vi "CRYFreq or Log Amp Sweep.vi"(4 "Output Flag":cluster{bool, bool, "ApplyEQ":bool}, 6 "Stimulus Para":T3={"Name"="", "Level Out"=0.9999999999999998, "Start Freq"=6300.0, "Stop Freq"=100.0, "Steps"=19, "Cycles"=12, "Sweep type"=0, "Freq"=1000.0, "Start ampl"=0.9999999999999998, "Stop ampl"=0.9999999999999998, "sine waves"=[], "wav path"="", "Sweep time"=0.9999999999999998, "Resolution"=0, "Tone type6"=0, "fix/ratio6"=0, "Ratio6"=0, "Difference6"=0, "RatioFreq6"=0} {"Resolution" items=["R10(1/3 Oct.)", "R20(1/6 Oct.)", "R40(1/12 Oct.)", "R80(1/24 Oct.)", "User Defined, Log", "User Defined,Linear"]; "Sweep time" format="%.2f"; "Stop ampl" format="%.2f"; "Start ampl" format="%.2f"; "Freq" format="%.2f"; "sine waves"."cycles" format="%.2f"; "sine waves"."ampl" format="%.2f"; "sine waves"."freq" format="%.2f"; "Level Out" format="%.2f"}, 7 "end":bool, 8 "FAPS in":T4(array[cluster]) {"cycles" format="%.2f"; "ampl" format="%.2f"; "freq" format="%.2f"}, 9 "Master sine waves":cluster{"freq":dbl, "ampl":dbl, "cycles":dbl}[](array[cluster]) {"cycles" format="%.2f"; "ampl" format="%.2p"; "freq" format="%.2f"}, 10 "EQ Curve":T1={"Name"="", "Curve"=[], "X data"=1, "Y data"=1, "Z data"=1, "X axis"=0, "Y axis"=1, "Z axis"=1, "X unit"="Hz", "Y unit"="", "Z unit"="deg.", "X dB ref"=1.0, "Y dB ref"=1.0, "Z dB ref"=1.0, "single val"=FALSE, "protected"=FALSE, "display X"=TRUE, "display Y"=TRUE, "display Z"=TRUE, "Test Info"="", "Step No."=0, "Plot Settings"={"Color"=0, "Interpolation"=0, "Point Style"=0, "Line Style"=0, "Point Color"=0, "Line Width"=0, "Bar Plot Style"=0, "Fill To"=0}, "AutoProtect"=FALSE} {"Z data" items=["dB", "Lin"]; "X data" items=["dB", "Lin"]; "Y data" items=["dB", "Lin"]; "Z dB ref" format="%.1f"; "Z axis" items=["Log", "Lin"]; "X dB ref" format="%.1f"; "X axis" items=["Log", "Lin"]; "Y axis" items=["Log", "Lin"]; "Y dB ref" format="%.1f"; "Curve"."z" format="%.2f"; "Curve"."y" format="%.2f"; "Curve"."x" format="%.2f"}, 11 "Param1":T2) -> (1 "FAPS out":T4(array[cluster]) {"cycles" format="%.2f"; "ampl" format="%.2f"; "freq" format="%.2f"}, 2 "Stimulus out":sgl[](array[numeric]), 3 "Diff Frequency":dbl)   [LabVIEW 2013]
uses:
  Typedef Control/CRYStimulus Parameter.ctl
  Typedef Control/CRYData Cluster.ctl
  <vilib>/Analysis/NI_AALBase.lvlib
panel:
  out "x/y":dbl format="%#_6p"
  out "Waveform Graph":waveform(sgl)(graph)
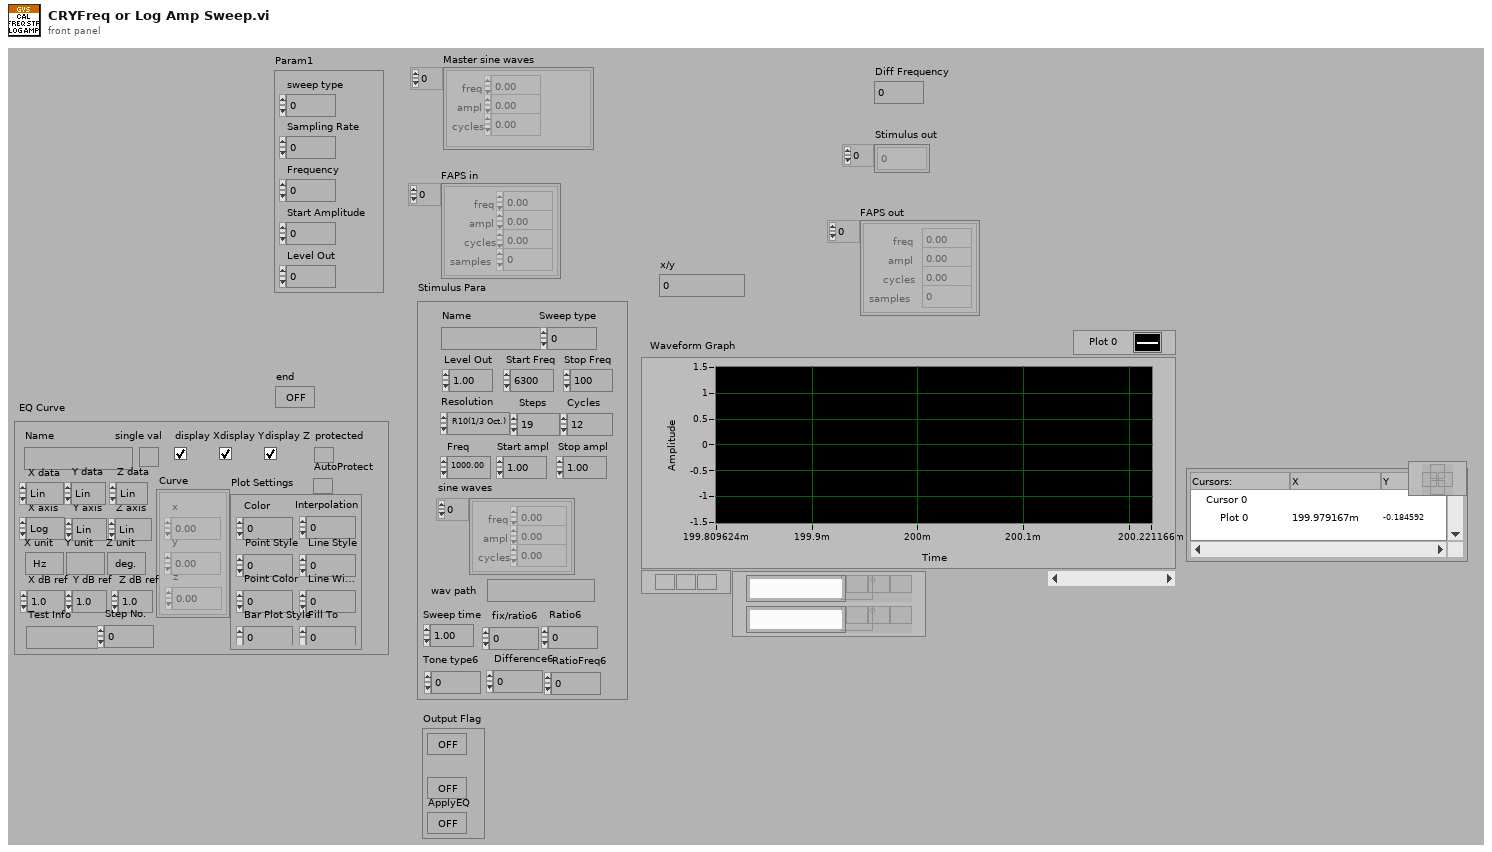
[diagram p1: front panel]
types:
  T1 = typedef "CRYData Cluster.ctl" = cluster{"Name":string, "Curve":cluster{"x":dbl, "y":dbl, "z":dbl}[], "X data":u16, "Y data":u16, "Z data":u16, "X axis":u16, "Y axis":u16, "Z axis":u16, "X unit":string, "Y unit":string, "Z unit":string, "X dB ref":dbl, "Y dB ref":dbl, "Z dB ref":dbl, "single val":bool, "protected":bool, "display X":bool, "display Y":bool, "display Z":bool, "Test Info":string, "Step No.":i32, "Plot Settings":cluster{"Color":u32, "Interpolation":u8, "Point Style":u8, "Line Style":u8, "Point Color":u32, "Line Width":u8, "Bar Plot Style":u8, "Fill To":i16}, "AutoProtect":bool}
  T2 = cluster{"sweep type":i32, "Sampling Rate":dbl, "Frequency":dbl, "Start Amplitude":dbl, "Level Out":dbl}
  T3 = typedef "CRYStimulus Parameter.ctl" = cluster{"Name":string, "Level Out":dbl, "Start Freq":dbl, "Stop Freq":dbl, "Steps":u32, "Cycles":u32, "Sweep type":i32, "Freq":dbl, "Start ampl":dbl, "Stop ampl":dbl, "sine waves":cluster{"freq":dbl, "ampl":dbl, "cycles":dbl}[], "wav path":string, "Sweep time":dbl, "Resolution":u16, "Tone type6":u16, "fix/ratio6":u16, "Ratio6":u16, "Difference6":u32, "RatioFreq6":u32}
  T4 = cluster{"freq":dbl, "ampl":dbl, "cycles":dbl, "samples":i32}[]
  T5 = cluster{"freq":dbl, "ampl":dbl, "cycles":dbl, "samples":i32}
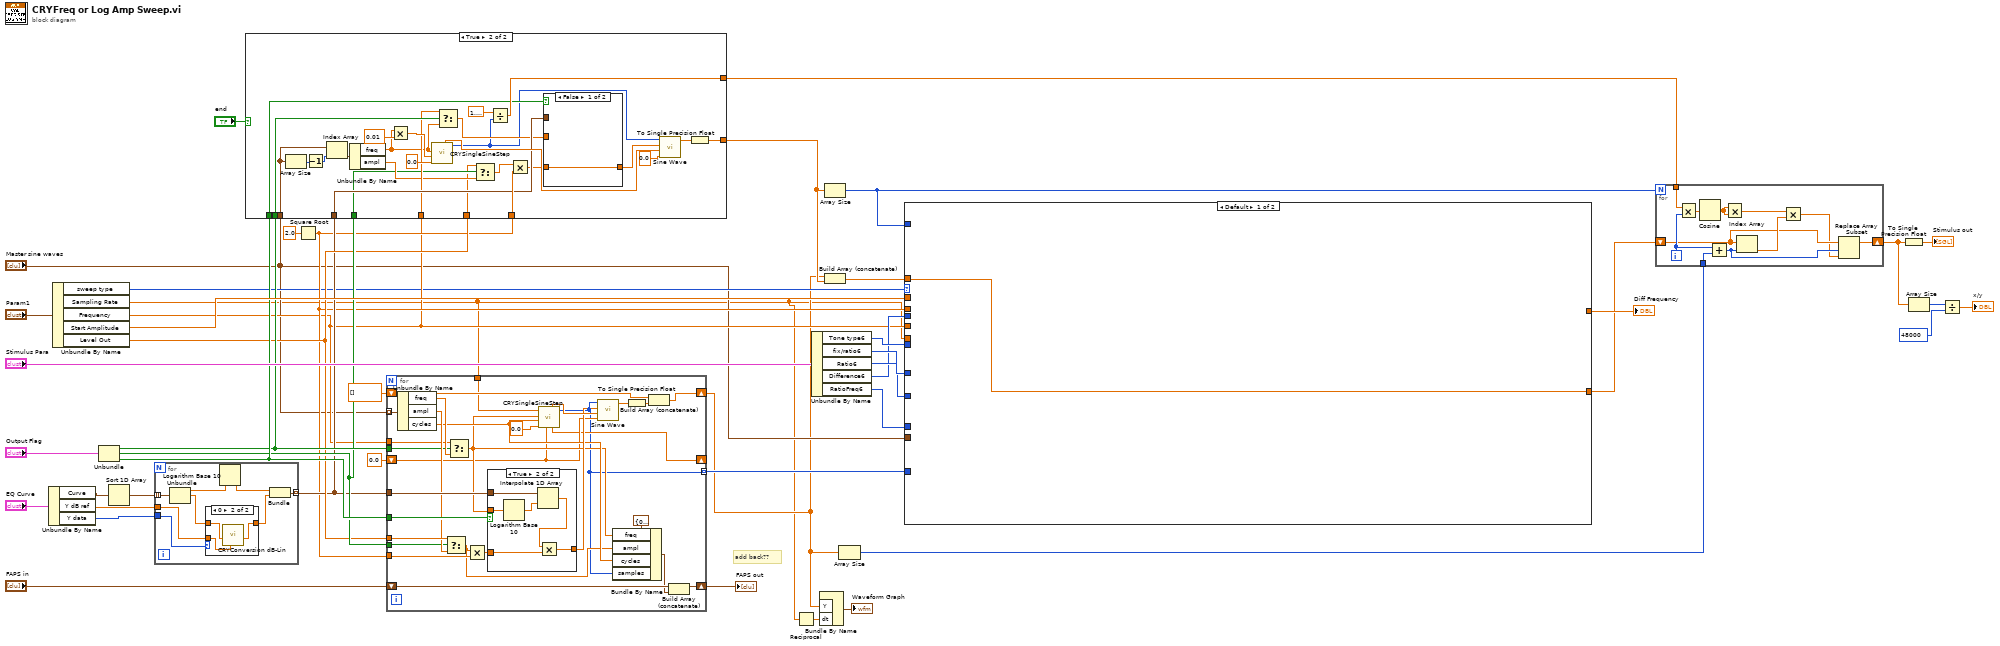
[diagram p0: block diagram]
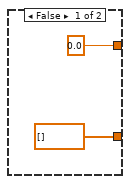
[diagram p2: hidden frame]
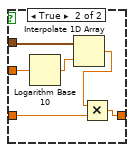
[diagram p3: hidden frame]
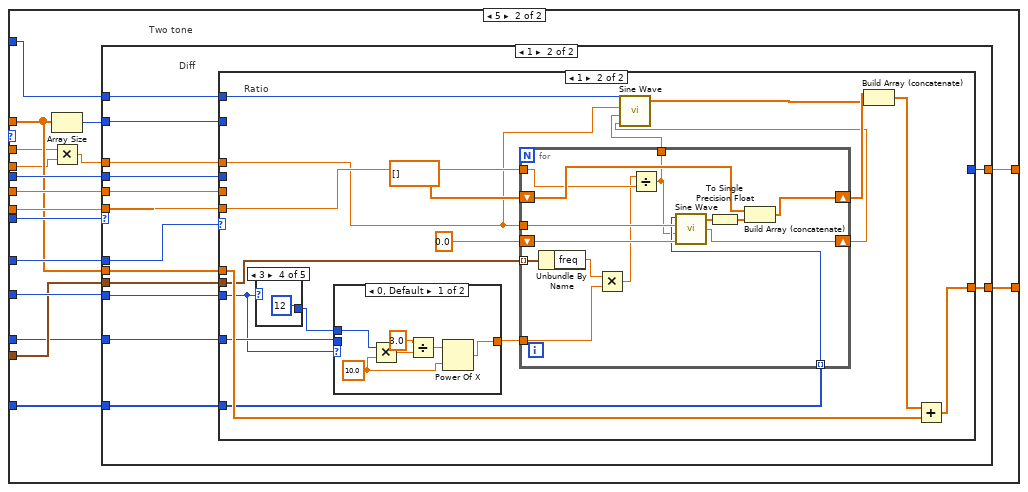
[diagram p6: hidden frame]
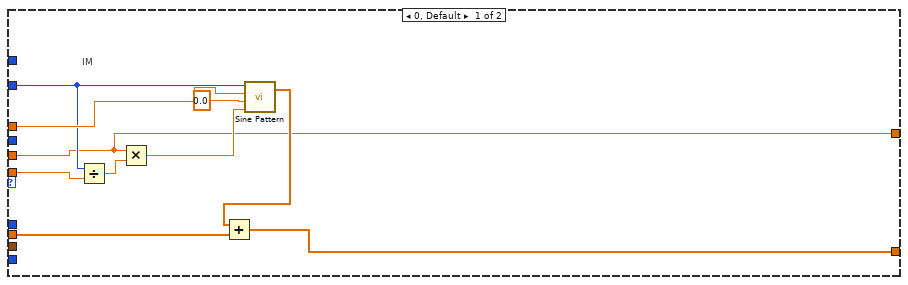
[diagram p7: hidden frame]
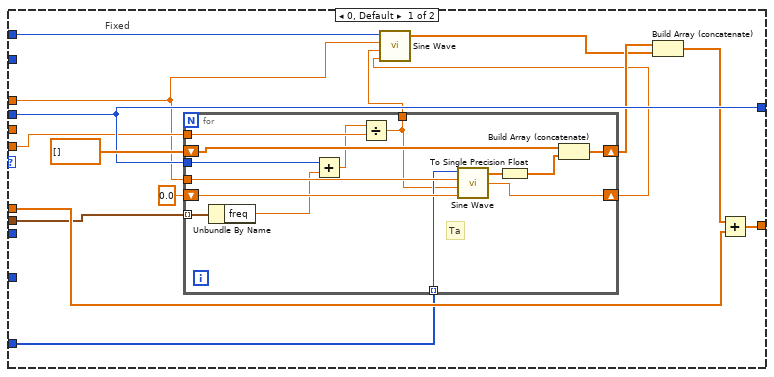
[diagram p8: hidden frame]
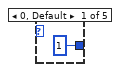
[diagram p9: hidden frame]
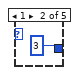
[diagram p10: hidden frame]
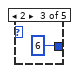
[diagram p11: hidden frame]
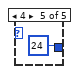
[diagram p12: hidden frame]
diagram:
  # "add back??"
  n1 = Unbundle By Name("EQ Curve") -> ("Curve"=w23:cluster{"x":dbl, "y":dbl, "z":dbl}[], "Y dB ref"=w22:dbl, "Y data"=w21:u16)
  n2 = Unbundle By Name("Param1") -> ("sweep type"=w10:i32, "Sampling Rate"=w6:dbl, "Frequency"=w13:dbl, "Start Amplitude"=w32:dbl, "Level Out"=w26:dbl)
  n3 = Unbundle("Output Flag") -> (w28:bool, w27:bool, "ApplyEQ"=w29:bool)
  n4 = Sort 1D Array(array=w23) -> (sorted array=w35:cluster{"x":dbl, "y":dbl, "z":dbl}[])
  n5 = for {
    tunnel: w35 -> [w54] mode=indexing
    tunnel: [w52] -> w20 mode=indexing
    tunnel: w22 -> [w50]
    tunnel: w21 -> [w49]
    n6 = Unbundle(w54) -> ("x"=w48:dbl, "y"=w47:dbl)  [unwired: 1 out]
    n7 = case shown="0" w49 {
      tunnel: w47 -> [w55 w58]
      tunnel: [w55 w57] -> w51
      tunnel: w50 -> [_ w56]
      frame 1, Default {
      }
      frame 0 {
        n8 = call "CRYConversion dB-Lin.vi"("dB ref."=w56, "Log In"=w58) -> ("Lin Out"=w57:dbl)  [unwired: 4 in, 3 out]
      }
    }
    n9 = Logarithm Base 10(1:w48) -> (0:w53:dbl)
    n10 = Bundle(w53, "Lin Out"=w51) -> (w52:cluster{dbl, "Lin Out":dbl})  [unwired: 1 out]
  }
  n11 = Square Root(x=2.0) -> (sqrt(x)=w14:dbl)
  n12 = case shown="True" "end" {
    tunnel: "Master sine waves" -> [_ w77]
    tunnel: [0.0 w76] -> w31
    tunnel: w14 -> [_ w75]
    tunnel: w29 -> [_ w74]
    tunnel: w20 -> [_ w73]
    tunnel: w28 -> [_ w72]
    tunnel: w13 -> [_ w70]
    tunnel: [sgl[] [] w69] -> w16
    tunnel: w27 -> [_ w64]
    tunnel: w26 -> [_ w63]
    frame False {
    }
    frame True {
      n13 = Array Size(array=w77) -> (size(s)=w87:i32)
      n14 = Decrement(x=w87) -> (x-1=w86:i32)
      n15 = Index Array(array=w77, index=w86) -> (element=w85:cluster{"freq":dbl, "ampl":dbl, "cycles":dbl})
      n16 = Unbundle By Name(w85) -> ("freq"=w61:dbl, "ampl"=w66:dbl)
      n17 = Multiply(x=w61, y=0.01) -> (x*y=w79:dbl)
      n18 = call "CRYSingleSineStep.vi"("Freq"=w61, "Cycles per freq"=w79, "Cycles discarded"=0.0) -> ("RelFreq"=w83:dbl, "TotalSamples"=w62:i32)  [unwired: 2 in, 4 out]
      n19 = Select(t=w70, s=w72, f=w61) -> (s? t:f=w71:dbl)
      n20 = Select(t=w63, s=w64, f=w66) -> (s? t:f=w65:dbl)
      n21 = Divide(x=1.5707963267948966, y=w62) -> (x/y=w76:dbl)
      n22 = Multiply(x=w65, y=w75) -> (x*y=w68:dbl)
      n23 = case shown="False" w74 {
        tunnel: [w88 w91] -> w67
        tunnel: w68 -> [w88 w94]
        tunnel: w73 -> [_ w92]
        tunnel: w71 -> [_ w89]
        frame False {
        }
        frame True {
          n24 = Logarithm Base 10(1:w89) -> (0:w90:dbl)
          n25 = Interpolate 1D Array(1:w90, 2:w92) -> (0:w93:dbl)
          n26 = Multiply(x=w93, y=w94) -> (x*y=w91:dbl)
        }
      }
      n27 = call <vilib>:"Sine Wave.vi"("samples"=w62, "amplitude"=w67, "frequency"=w83, "phase in"=0.0) -> ("sine wave"=w81:dbl[])  [unwired: 1 in, 2 out]
      n28 = To Single Precision Float(number=w81) -> (single precision float=w69:sgl[])
    }
  }
  n29 = for {
    shift-right: [w123] -> w8
    shift-left: sgl[] [] -> [w122]
    tunnel: w29 -> [w120]
    tunnel: w20 -> [w121]
    tunnel: "Master sine waves" -> [w119] mode=indexing
    tunnel: w14 -> [w118]
    tunnel: w6 -> [w110]
    tunnel: w26 -> [w116]
    tunnel: w13 -> [w111]
    shift-right: [w99] -> _
    shift-left: 0.0 -> [w100]
    shift-right: [w95] -> w39
    shift-left: "FAPS in" -> [w97]
    tunnel: w27 -> [w104]
    tunnel: w28 -> [w103]
    tunnel: [w98] -> w17 mode=indexing
    n30 = Unbundle By Name(w119) -> ("freq"=w115:dbl, "ampl"=w113:dbl, "cycles"=w106:dbl)
    n31 = Select(t=w116, s=w104, f=w113) -> (s? t:f=w102:dbl)
    n32 = Select(t=w111, s=w103, f=w115) -> (s? t:f=w101:dbl)
    n33 = Multiply(x=w102, y=w118) -> (x*y=w117:dbl)
    n34 = case shown="True" w120 {
      tunnel: [w124 w127] -> w107
      tunnel: w117 -> [w124 w130]
      tunnel: w121 -> [_ w128]
      tunnel: w101 -> [_ w126]
      frame False {
      }
      frame True {
        n35 = Logarithm Base 10(1:w126) -> (0:w125:dbl)
        n36 = Interpolate 1D Array(1:w125, 2:w128) -> (0:w129:dbl)
        n37 = Multiply(x=w129, y=w130) -> (x*y=w127:dbl)
      }
    }
    n38 = call "CRYSingleSineStep.vi"("Fs"=w110, "Freq"=w101, "Cycles per freq"=w106, "Cycles discarded"=0.0 ("phase in"), "StartPhase"=w100) -> ("RelFreq"=w108:dbl, "StopPhase"=w99:dbl, "TotalSamples"=w98:i32)  [unwired: 3 out]
    n39 = call <vilib>:"Sine Wave.vi"("samples"=w98, "amplitude"=w107, "frequency"=w108, "phase in"=w100) -> ("sine wave"=w114:dbl[])  [unwired: 1 in, 2 out]
    n40 = Bundle By Name(cluster=T5 {"freq"=0.0, "ampl"=0.0, "cycles"=0.0, "samples"=0}, "freq"=w101, "ampl"=w102, "cycles"=w106, "samples"=w98) -> (w96:T5)
    n41 = To Single Precision Float(number=w114) -> (single precision float=w109:sgl[])
    n42 = Build Array (concatenate)(w122, w109) -> (w123:sgl[])
    n43 = Build Array (concatenate)(w97, w96) -> (w95:T4)
  }
  "FAPS out" <- w39
  n44 = Reciprocal(x=w6) -> (1/x=w5:dbl)
  n45 = Unbundle By Name("Stimulus Para") -> ("Tone type6"=w46:u16, "fix/ratio6"=w45:u16, "Ratio6"=w44:u16, "Difference6"=w43:u32, "RatioFreq6"=w42:u32)
  n46 = Bundle By Name("Y"=w8, "dt"=w5) -> (→"Waveform Graph":waveform(sgl))  [unwired: 1 in]
  n47 = Build Array (concatenate)(w8, w16) -> (w19:sgl[])
  n48 = Array Size(array=w16) -> (size(s)=w18:i32)
  n49 = Array Size(array=w8) -> (size(s)=w30:i32)
  n50 = case shown="Default" w10 {
    tunnel: [w131 w148] -> w15
    tunnel: w43 -> [_ w142]
    tunnel: w46 -> [_ w147]
    tunnel: w45 -> [_ w146]
    tunnel: w44 -> [_ w145]
    tunnel: w6 -> [_ w144]
    tunnel: w13 -> [_ w143]
    tunnel: "Master sine waves" -> [_ w141]
    tunnel: w42 -> [_ w140]
    tunnel: [_ w139] -> w41
    tunnel: w19 -> [w131 w138]
    tunnel: w32 -> [_ w136]
    tunnel: w14 -> [_ w135]
    tunnel: w18 -> [_ w133]
    tunnel: w17 -> [_ w132]
    frame Default {
    }
    frame 5 {
      # "Two tone"
      n51 = Array Size(array=w138) -> (size(s)=w137:i32)
      n52 = Multiply(x=w136, y=w135) -> (x*y=w134:dbl)
      n53 = case shown="1" w147 {
        tunnel: w138 -> [w158 w172]
        tunnel: [w150 w171] -> w148
        tunnel: w137 -> [w153 w170]
        tunnel: w134 -> [w157 w169]
        tunnel: w146 -> [_ w168]
        tunnel: w145 -> [_ w167]
        tunnel: w144 -> [w151 w166]
        tunnel: w143 -> [w149 w165]
        tunnel: w142 -> [_ w164]
        tunnel: w141 -> [_ w159]
        tunnel: w140 -> [_ w163]
        tunnel: [w149 w162] -> w139
        tunnel: w133 -> [_ w161]
        tunnel: w132 -> [_ w160]
        frame 0, Default {
          # "IM"
          n54 = Divide(x=w153, y=w151) -> (x/y=w152:dbl)
          n55 = Multiply(x=w149, y=w152) -> (x*y=w154:dbl)
          n56 = call <vilib>:"Sine Pattern.vi"("cycles"=w154, "phase(degrees)"=0.0 ("phase in"), "amplitude"=w157, "samples"=w153) -> ("Sinusoidal Pattern"=w155:dbl[])  [unwired: 1 out]
          n57 = Add(x=w155, y=w158) -> (x+y=w150:dbl[])
        }
        frame 1 {
          # "Diff"
          n58 = case shown="1" w168 {
            tunnel: w172 -> [w185 w217]
            tunnel: [w176 w205] -> w171
            tunnel: w170 -> [_ _]
            tunnel: w169 -> [w175 w203]
            tunnel: w167 -> [_ w213]
            tunnel: w166 -> [w177 w210]
            tunnel: w165 -> [_ _]
            tunnel: w164 -> [w182 _]
            tunnel: w159 -> [w184 w204]
            tunnel: w163 -> [_ w214]
            tunnel: [w182 _] -> w162
            tunnel: w161 -> [w183 w209]
            tunnel: w160 -> [w180 w207]
            frame 0, Default {
              # "Fixed"
              n59 = for {
                tunnel: w175 -> [w201]
                tunnel: w184 -> [w200] mode=indexing
                shift-right: [w198] -> w174
                shift-left: 0.0 ("phase in") -> [w199]
                shift-right: [w195] -> w179
                shift-left: sgl[] [] -> [w196]
                tunnel: w182 -> [w197]
                tunnel: w177 -> [w192]
                tunnel: w180 -> [w189] mode=indexing
                tunnel: [w188] -> w173
                # "Ta"
                n60 = Unbundle By Name(w200) -> ("freq"=w191:dbl)
                n61 = Add(x=w197, y=w191) -> (x+y=w190:dbl)
                n62 = Divide(x=w190, y=w192) -> (x/y=w188:dbl)
                n63 = call <vilib>:"Sine Wave.vi"("samples"=w189, "amplitude"=w201, "frequency"=w188, "phase in"=w199) -> ("sine wave"=w194:dbl[], "phase out"=w198:dbl)  [unwired: 1 in, 1 out]
                n64 = To Single Precision Float(number=w194) -> (single precision float=w193:sgl[])
                n65 = Build Array (concatenate)(w196, w193) -> (w195:sgl[])
              }
              n66 = call <vilib>:"Sine Wave.vi"("samples"=w183, "amplitude"=w175, "frequency"=w173, "phase in"=w174) -> ("sine wave"=w178:dbl[])  [unwired: 1 in, 2 out]
              n67 = Build Array (concatenate)(w179, w178) -> (w181:dbl[])
              n68 = Add(x=w181, y=w185) -> (x+y=w176:dbl[])
            }
            frame 1 {
              # "Ratio"
              n69 = case shown="3" w213 {
                tunnel: [u16 1 ("y") u16 3 ("y") u16 6 ("y") u16 12 ("y") u16 24 ("y")] -> w215
                frame 0, Default {
                }
                frame 1 {
                }
                frame 2 {
                }
                frame 3 {
                }
                frame 4 {
                }
              }
              n70 = case shown="0, Default" w213 {
                tunnel: w214 -> [_ w231]
                tunnel: [w226 w231] -> w216
                tunnel: w215 -> [w225 _]
                frame 0, Default {
                  w227 = 10.0 ("x")
                  n71 = Multiply(x=w225, y=w227) -> (x*y=w228:dbl)
                  n72 = Divide(x=3.0, y=w228) -> (x/y=w229:dbl)
                  n73 = Power Of X(1:w227, 2:w229) -> (0:w226:dbl)
                }
                frame 5 {
                }
              }
              n74 = for {
                tunnel: w203 -> [w245]
                tunnel: w204 -> [w244] mode=indexing
                shift-right: [w242] -> w208
                shift-left: 0.0 ("phase in") -> [w243]
                shift-right: [w240] -> w212
                shift-left: sgl[] [] -> [w241]
                tunnel: w210 -> [w237]
                tunnel: w216 -> [w235]
                tunnel: w207 -> [w233] mode=indexing
                tunnel: [w232] -> w202
                n75 = Unbundle By Name(w244) -> ("freq"=w236:dbl)
                n76 = Multiply(x=w236, y=w235) -> (x*y=w234:dbl)
                n77 = Divide(x=w234, y=w237) -> (x/y=w232:dbl)
                n78 = call <vilib>:"Sine Wave.vi"("samples"=w233, "amplitude"=w245, "frequency"=w232, "phase in"=w243) -> ("sine wave"=w239:dbl[], "phase out"=w242:dbl)  [unwired: 1 in, 1 out]
                n79 = To Single Precision Float(number=w239) -> (single precision float=w238:sgl[])
                n80 = Build Array (concatenate)(w241, w238) -> (w240:sgl[])
              }
              n81 = call <vilib>:"Sine Wave.vi"("samples"=w209, "amplitude"=w203, "frequency"=w202, "phase in"=w208) -> ("sine wave"=w211:dbl[])  [unwired: 1 in, 2 out]
              n82 = Build Array (concatenate)(w212, w211) -> (w206:dbl[])
              n83 = Add(x=w206, y=w217) -> (x+y=w205:dbl[])
            }
          }
        }
      }
    }
  }
  "Diff Frequency" <- w41
  n84 = for {
    N: w18 -> [_]
    tunnel: w31 -> [w253]
    tunnel: w30 -> [w252]
    shift-right: [w246] -> w4
    shift-left: w15 -> [w248]
    i -> [w251]
    n85 = Multiply(x=w253, y=w251) -> (x*y=w256:dbl)
    n86 = Cosine(x=w256) -> (cos(x)=w255:dbl)
    n87 = Add(x=w251, y=w252) -> (x+y=w250:i32)
    n88 = Multiply(x=w255, y=w255) -> (x*y=w254:dbl)
    n89 = Index Array(array=w248, index=w250) -> (element=w249:dbl)
    n90 = Multiply(x=w254, y=w249) -> (x*y=w247:dbl)
    n91 = Replace Array Subset(array=w248, new element=w247, index=w250) -> (w246:dbl[])
  }
  n92 = To Single Precision Float(number=w4) -> (single precision float=→"Stimulus out":sgl[])
  n93 = Array Size(array=w4) -> (size(s)=w3:i32)
  n94 = Divide(x=w3, y=48000) -> (x/y=→"x/y":dbl)
